vi "display_for_end_record.vi"(8 "error in":errorcluster) -> (0 "error out":errorcluster)   [LabVIEW 2016]
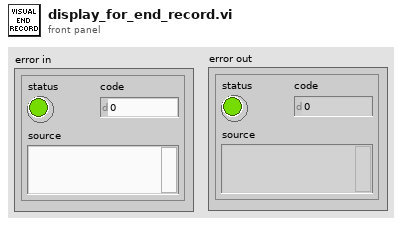
[diagram p1: front panel]
types:
  T1 = enum8{"Enabled", "Disabled", "Disabled and Grayed Out"}
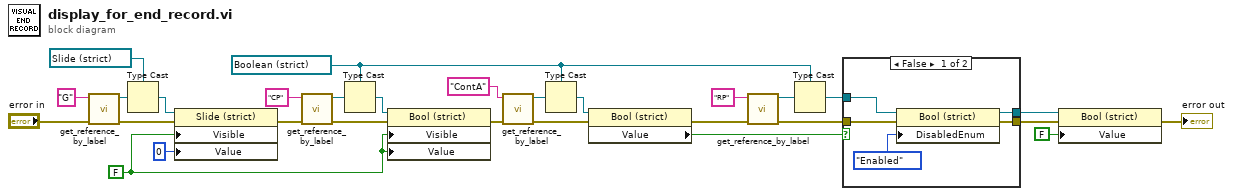
[diagram p0: block diagram]
diagram:
  w14 = refnum<vi> refnum ("ContA")
  w29 = FALSE ("Visible")
  n1 = call "get_reference_by_label.vi"("error in"="error in", "Label"="G") -> ("error out"=w26:errorcluster, "Ctl Refnum"=w13:refnum<vi>)  [unwired: 7 in, 1 out]
  n2 = Type Cast(type=refnum<vi> refnum ("G"), x=w13) -> (*(type *) &x=w11:refnum<vi>)
  n3 = property on="Property Node" class="Slide (strict)"(reference=w11, error in=w26, "Visible"=w29, "Value"=u8 0) -> (error out=w24:errorcluster)  [unwired: 1 out]
  n4 = call "get_reference_by_label.vi"("error in"=w24, "Label"="CP") -> ("error out"=w23:errorcluster, "Ctl Refnum"=w22:refnum<vi>)  [unwired: 7 in, 1 out]
  n5 = Type Cast(type=w14, x=w22) -> (*(type *) &x=w21:refnum<vi>)
  n6 = property on="Property Node" class="Bool (strict)"(reference=w21, error in=w23, "Visible"=w29, "Value"=w29) -> (error out=w19:errorcluster)  [unwired: 1 out]
  n7 = call "get_reference_by_label.vi"("error in"=w19, "Label"="ContA") -> ("error out"=w16:errorcluster, "Ctl Refnum"=w18:refnum<vi>)  [unwired: 7 in, 1 out]
  n8 = Type Cast(type=w14, x=w18) -> (*(type *) &x=w17:refnum<vi>)
  n9 = property class="Bool (strict)"(reference=w17, error in=w16) -> (error out=w15:errorcluster, "Value"=w2:bool)  [unwired: 1 out]
  n10 = call "get_reference_by_label.vi"("error in"=w15, "Label"="RP") -> ("error out"=w8:errorcluster, "Ctl Refnum"=w7:refnum<vi>)  [unwired: 7 in, 1 out]
  n11 = Type Cast(type=w14, x=w7) -> (*(type *) &x=w6:refnum<vi>)
  n12 = case shown="False" w2 {
    tunnel: w8 -> [w33 w36]
    tunnel: w6 -> [w32 w35]
    tunnel: [w31 w36] -> w5
    tunnel: [w30 w35] -> w3
    frame False {
      n13 = property on="Property Node" class="Bool (strict)"(reference=w32, error in=w33, "DisabledEnum"=T1."Enabled" ("Disabled")) -> (reference out=w30:refnum<vi>, error out=w31:errorcluster)
    }
    frame True {
    }
  }
  n14 = property on="Property Node" class="Bool (strict)"(reference=w3, error in=w5, "Value"=FALSE) -> (error out=→"error out":errorcluster)  [unwired: 1 out]
